vi "[SubVI]Power_Assistance_L.vi"(2 "Left Torque Profile":dbl[](array[numeric]), 3 "ext onset":dbl=90.0 format="%#_13g", 4 "flex onset":dbl=45.0 format="%#_13g", 5 "Left Gait Phase":dbl format="%#_13g") -> (1 "Left Desired Torque":dbl)   [LabVIEW 2018]
uses:
  <vilib>/functionblocks/Edge Detection/One Shot Rising with Input/One Shot Rising with Input.vi
  <vilib>/functionblocks/FB Core/FB Core.xnode
  <vilib>/functionblocks/NI_FunctionBlock Libraries.lvlib
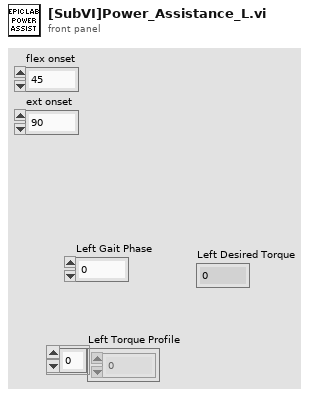
[diagram p1: front panel]
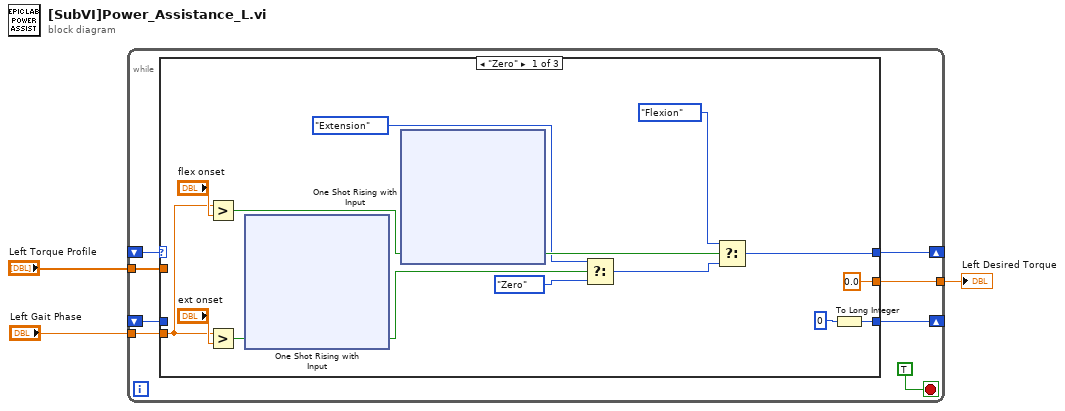
[diagram p0: block diagram]
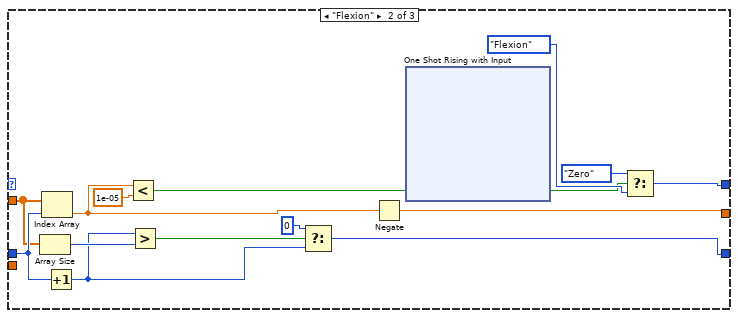
[diagram p2: hidden frame]
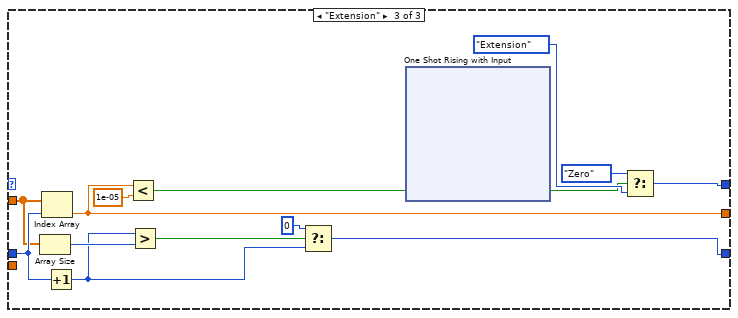
[diagram p3: hidden frame]
diagram:
  n1 = while {
    shift-right: [w10] -> _
    shift-left: _ -> [w9]
    tunnel: [w8] -> w1
    shift-right: [w6] -> _
    shift-left: _ -> [w7]
    tunnel: "Left Torque Profile" -> [w5]
    tunnel: "Left Gait Phase" -> [w4]
    stop <- TRUE stop-if-true
    n2 = case shown="\"Zero\"" w7 {
      tunnel: w9 -> [_ w116 w166]
      tunnel: [w23 w107 w159] -> w10
      tunnel: w5 -> [_ w112 w162]
      tunnel: [0.0 ("Numeric") w103 w156] -> w8
      tunnel: w4 -> [w14 _ _]
      tunnel: [w22 w117 w165] -> w6
      frame "Zero" {
        n3 = Greater?(x=w14, y="flex onset") -> (0:w20:bool)
        n4 = Greater?(x=w14, y="ext onset") -> (0:w13:bool)
        n5 = xnode "One Shot Rising with Input"("input"=w13) -> ("output"=w17:bool)  [unwired: 1 in, 1 out]
        n6 = xnode "One Shot Rising with Input"("input"=w20) -> ("output"=w19:bool)  [unwired: 1 in, 1 out]
        n7 = Select(t=enum16{"Extension", "Zero", "Flexion"}."Extension", s=w17, f=enum16{"Extension", "Zero", "Flexion"}."Zero") -> (s? t:f=w12:enum16{"Extension", "Zero", "Flexion"})
        n8 = Select(t=enum16{"Extension", "Zero", "Flexion"}."Flexion", s=w19, f=w12) -> (s? t:f=w22:enum16{"Extension", "Zero", "Flexion"})
        n9 = To Long Integer(number=u8 0) -> (32bit integer=w23:i32)
      }
      frame "Flexion" {
        n10 = Array Size(array=w112) -> (size(s)=w111:i32)
        n11 = Index Array(array=w112, index=w116) -> (element=w104:dbl)
        n12 = Increment(x=w116) -> (x+1=w108:i32)
        n13 = Less?(x=w104, y=1e-05) -> (x < y?=w105:bool)
        n14 = Greater?(x=w108, y=w111) -> (0:w110:bool)
        n15 = Select(t=0, s=w110, f=w108) -> (s? t:f=w107:i32)
        n16 = Negate(x=w104) -> (-x=w103:dbl)
        n17 = xnode "One Shot Rising with Input"("input"=w105) -> ("output"=w106:bool)  [unwired: 1 in, 1 out]
        n18 = Select(t=enum16{"Extension", "Zero", "Flexion"}."Zero", s=w106, f=enum16{"Extension", "Zero", "Flexion"}."Flexion") -> (s? t:f=w117:enum16{"Extension", "Zero", "Flexion"})
      }
      frame "Extension" {
        n19 = Array Size(array=w162) -> (size(s)=w161:i32)
        n20 = Index Array(array=w162, index=w166) -> (element=w156:dbl)
        n21 = Increment(x=w166) -> (x+1=w160:i32)
        n22 = Less?(x=w156, y=1e-05) -> (x < y?=w158:bool)
        n23 = Greater?(x=w160, y=w161) -> (0:w164:bool)
        n24 = Select(t=0, s=w164, f=w160) -> (s? t:f=w159:i32)
        n25 = xnode "One Shot Rising with Input"("input"=w158) -> ("output"=w157:bool)  [unwired: 1 in, 1 out]
        n26 = Select(t=enum16{"Extension", "Zero", "Flexion"}."Zero", s=w157, f=enum16{"Extension", "Zero", "Flexion"}."Extension") -> (s? t:f=w165:enum16{"Extension", "Zero", "Flexion"})
      }
    }
  }
  "Left Desired Torque" <- w1
